vi "FTW-Ether-CreateClient.vi"(5 "Server Address":T1, 11 "error in":errorcluster) -> (4 "Client Endpoint":refnum<class "FTW-Endpoint.lvclass">, 15 "error out":errorcluster)   [LabVIEW 2012, in "FTW-Actor.lvlib" / "FTW-Ether.lvclass"]
uses:
  FTW-Ether.lvclass
  Endpoint/FTW-Endpoint.lvclass
  Utility/FTW-Actor-Address.ctl
  FTW-Ether-EndpointType.ctl
  FTW-Actor.lvlib
panel:
  # "Inputs"
  # "Outputs"
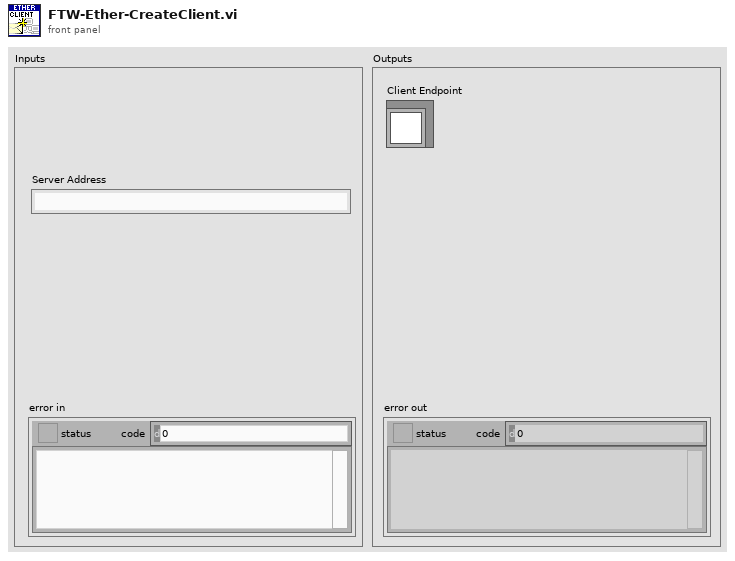
[diagram p1: front panel]
types:
  T1 = typedef "FTW-Actor.lvlib/FTW-Actor-Address.ctl" = string
  T2 = typedef "FTW-Actor.lvlib/FTW-Ether.lvclass/FTW-Ether-EndpointType.ctl" = enum16{"Server", "Client", "Publisher", "Subscriber"}
  T3 = typedef "FTW-Actor.lvlib/FTW-Ether.lvclass/FTW-Ether-MessageTransportScheme.ctl" = enum16{"ØMQ TCP (tcp://)", "ØMQ In-Process (inproc://)", "LabVIEW Queues (lvq://)", "LabVIEW Network Streams (lvns://)"}
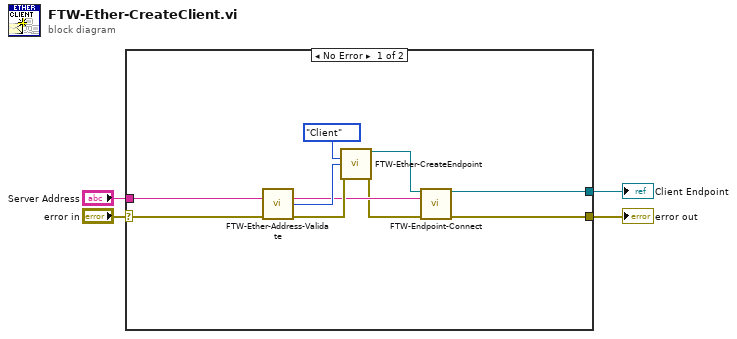
[diagram p0: block diagram]
diagram:
  n1 = case shown="No Error" "error in" {
    selector: "error in" -> [w11 w15]
    tunnel: [w14 _] -> w1
    tunnel: [w13 w15] -> w2
    tunnel: "Server Address" -> [w10 _]
    frame No Error {
      n2 = call "FTW-Ether-Address-Validate.vi"("Address"=w10, "error in"=w11) -> ("Sanitized Address"=w8:T1, "Message Transport Scheme"=w9:T3, "error out"=w12:errorcluster)  [unwired: 11 in]
      n3 = call "FTW-Ether-CreateEndpoint.vi"("Endpoint Type"=FTW-Ether-EndpointType."Client", "Message Transport Scheme"=w9, "error in"=w12) -> ("FTW Endpoint"=w7:refnum<class "FTW-Endpoint.lvclass">, "error out"=w5:errorcluster)  [unwired: 11 in]
      n4 = call-dynamic "FTW-Endpoint-Connect.vi"("FTW Endpoint Type"=w7, "Endpoint Address"=w8, "error in"=w5) -> ("FTW Endpoint"=w14:refnum<class "FTW-Endpoint.lvclass">, "error out"=w13:errorcluster)  [unwired: 11 in]
    }
    frame Error {
    }
  }
  "error out" <- w2
  "Client Endpoint" <- w1
